vi "Get_Data_With_Condition.vi"(8 "error in (no error)":errorcluster caption="entrée d'erreur (pas d'erreur)", 11 "Firebase Benches en entrée":refnum<class "Firebase Packaging_ListProduct.lvclass">) -> (0 "error out":errorcluster caption="sortie d'erreur", 3 "Firebase Benches en sortie":refnum<class "Firebase Packaging_ListProduct.lvclass">)   [LabVIEW 2020, in "Library Instrument & Equipement.lvlib" / "Library FireBase.lvlib" / "Firebase Packaging_ListProduct.lvclass"]
doc: "Returns data according to Value_To_Find on Collection_to_find Use Nb_To_Read to determine the number to read\nPlease initialise the following values before use the VI\n - Name BDD\n - Value to find\n - API Key\n - Field Filter\n - Field Order\n - Collection_to_find\n\nIf there is no Field order -> Field Order=Field Filter"
uses:
  Firebase Packaging_ListProduct.lvclass
  C:/Users/ngarcin/OneDrive - Altyor/Standard TB/Class/Firebase/Source/Firebase Driver/Firebase Driver.lvclass
  C:/Users/ngarcin/OneDrive - Altyor/Standard TB/Class/Firebase/Source/Firebase Packaging/Firebase Packaging.lvclass
  JSON API/JSON Value/Set from JSON string.vi
  JSON API/JSON Value/JSON Value.lvclass
  Firebase Packaging_ListProduct.lvclass/Firebase Packaging_ListProduct.ctl
  JSON API/Variant JSON/Variant JSON.lvlib
  JSON API/Get Polymorphic/JSON GetSet.lvlib
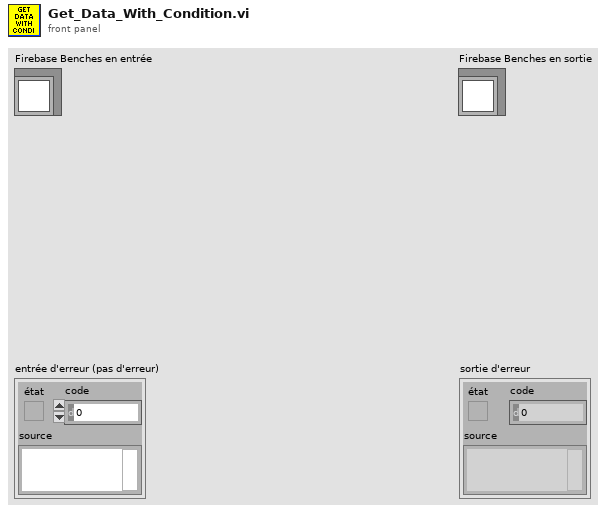
[diagram p1: front panel]
types:
  T1 = cluster{"documents":cluster{"name":string, "fields":cluster{"Result":cluster{"booleanValue":bool}, "CreationDate":cluster{"timestampValue":string}, "Batch":cluster{"stringValue":string}, "SerialNumber":cluster{"stringValue":string}, "EndOfProduction":cluster{"timestampValue":string}, "PartNumber":cluster{"stringValue":string}, "OrderNumber":cluster{"stringValue":string}, "Operator":cluster{"stringValue":string}}}[]}
  T2 = cluster{"name":string, "fields":cluster{"Result":cluster{"booleanValue":bool}, "CreationDate":cluster{"timestampValue":string}, "Batch":cluster{"stringValue":string}, "SerialNumber":cluster{"stringValue":string}, "EndOfProduction":cluster{"timestampValue":string}, "PartNumber":cluster{"stringValue":string}, "OrderNumber":cluster{"stringValue":string}, "Operator":cluster{"stringValue":string}}}[]
  T3 = cluster{"name":string, "fields":cluster{"Result":cluster{"booleanValue":bool}, "CreationDate":cluster{"timestampValue":string}, "Batch":cluster{"stringValue":string}, "SerialNumber":cluster{"stringValue":string}, "EndOfProduction":cluster{"timestampValue":string}, "PartNumber":cluster{"stringValue":string}, "OrderNumber":cluster{"stringValue":string}, "Operator":cluster{"stringValue":string}}}
  T4 = cluster{"document":cluster{"name":string, "fields":cluster{"Result":cluster{"booleanValue":bool}, "CreationDate":cluster{"timestampValue":string}, "Batch":cluster{"stringValue":string}, "SerialNumber":cluster{"stringValue":string}, "EndOfProduction":cluster{"timestampValue":string}, "PartNumber":cluster{"stringValue":string}, "OrderNumber":cluster{"stringValue":string}, "Operator":cluster{"stringValue":string}}}}
  T5 = cluster{"document":cluster{"name":string, "fields":cluster{"Result":cluster{"booleanValue":bool}, "CreationDate":cluster{"timestampValue":string}, "Batch":cluster{"stringValue":string}, "SerialNumber":cluster{"stringValue":string}, "EndOfProduction":cluster{"timestampValue":string}, "PartNumber":cluster{"stringValue":string}, "OrderNumber":cluster{"stringValue":string}, "Operator":cluster{"stringValue":string}}}}[]
  T6 = cluster{cluster{"name":string, "fields":cluster{"Result":cluster{"booleanValue":bool}, "CreationDate":cluster{"timestampValue":string}, "Batch":cluster{"stringValue":string}, "SerialNumber":cluster{"stringValue":string}, "EndOfProduction":cluster{"timestampValue":string}, "PartNumber":cluster{"stringValue":string}, "OrderNumber":cluster{"stringValue":string}, "Operator":cluster{"stringValue":string}}}[]}
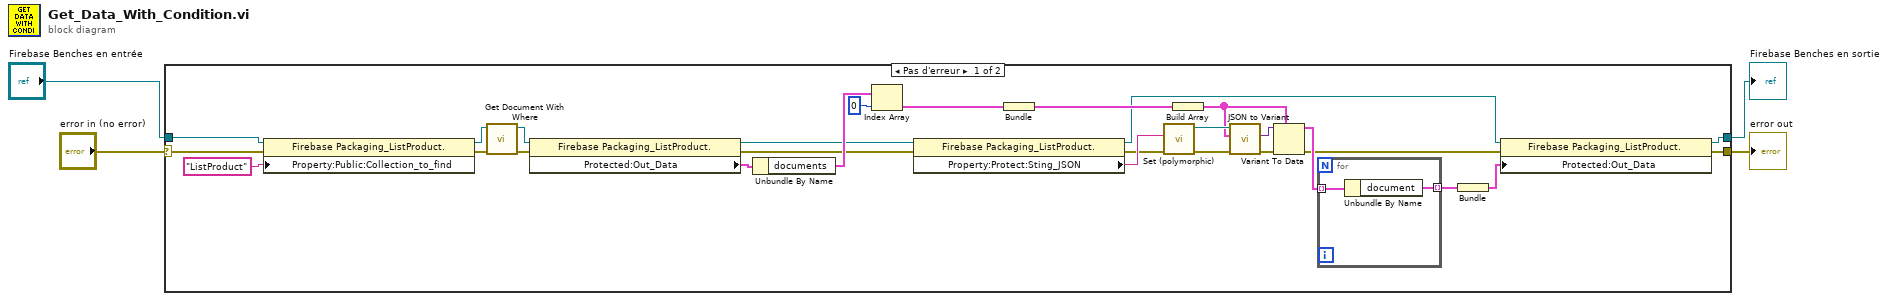
[diagram p0: block diagram]
diagram:
  n1 = case shown="Pas d'erreur" "error in (no error)" {
    selector: "error in (no error)" -> [w20 w36]
    tunnel: "Firebase Benches en entrée" -> [w21 w35]
    tunnel: [w8 w36] -> w3
    tunnel: [w15 w35] -> w2
    frame No Error {
      n2 = property class="Firebase Packaging_ListProduct."(reference=w21, error in=w20, "Property:Public:Collection_to_find"="ListProduct" ("Collection_to_find")) -> (reference out=w17:refnum<class "Firebase Packaging_ListProduct.lvclass">, error out=w18:errorcluster)
      n3 = call-dynamic "Get Document With Where.vi"("error in (no error)"=w18, "Firebase (Default) en entrée"=w17) -> ("error out"=w7:errorcluster, "Firebase (Default) en sortie"=w14:refnum<class "Firebase Packaging_ListProduct.lvclass">)  [unwired: 8 in]
      n4 = property class="Firebase Packaging_ListProduct."(reference=w14, error in=w7) -> (reference out=w5:refnum<class "Firebase Packaging_ListProduct.lvclass">, error out=w6:errorcluster, "Protected:Out_Data"=w13:T1)
      n5 = Unbundle By Name(w13) -> ("documents"=w12:T2)
      n6 = Index Array(array=w12, index=0 ("indice")) -> (element=w27:T3)
      n7 = property class="Firebase Packaging_ListProduct."(reference=w5, error in=w6) -> (reference out=w16:refnum<class "Firebase Packaging_ListProduct.lvclass">, error out=w23:errorcluster, "Property:Protect:Sting_JSON"=w29:string)
      n8 = Bundle("document"=w27) -> (w26:T4)  [unwired: 1 in]
      n9 = call-poly "Set (polymorphic).vi"("error in (no error)"=w23, "JSON stream"=w29) -> ("error out"=w30:errorcluster, "JSON Value out"=w32:refnum<class "JSON Value.lvclass">)  [unwired: 7 in, 1 out]
      n10 = Build Array(w26) -> (w25:T5)
      n11 = call "JSON to Variant.vi"("error in (no error)"=w30, "Variant (Data Type)"=w25, "JSON Value"=w32) -> ("error out"=w31:errorcluster, "Variant out"=w22:variant)  [unwired: 7 in]
      n12 = Variant To Data(error in=w31, type=w25, Variant=w22) -> (data=w24:T5, error out=w9:errorcluster)
      n13 = for {
        tunnel: w24 -> [w34] mode=indexing
        tunnel: [w33] -> w11 mode=indexing
        n14 = Unbundle By Name(w34) -> ("document"=w33:T3)
      }
      n15 = Bundle(w11) -> (w10:T6)  [unwired: 1 in]
      n16 = property class="Firebase Packaging_ListProduct."(reference=w16, error in=w9, "Protected:Out_Data"=w10) -> (reference out=w15:refnum<class "Firebase Packaging_ListProduct.lvclass">, error out=w8:errorcluster)
    }
    frame Error {
    }
  }
  "error out" <- w3
  "Firebase Benches en sortie" <- w2
